vi "SetAttributeViBoolean.vi"(7 "AttributeValue (Off)":bool, 8 "error in (no error)":errorcluster {"code" format="%.0x"}, 9 "AttributeID":u32(ring)=1150001 items=["CHANNEL_AVERAGING"=1150001, "CHANNEL_CORRECTION"=1150003, "CHANNEL_MEASUREMENT_LIMIT_ENABLE"=1150018, "CHANNEL_MEASUREMENT_MARKER_ENABLED"=1150022, "CHANNEL_MEASUREMENT_MARKER_MARKER_TRACK_ENABLED"=1150023, "CHANNEL_MEASUREMENT_SMOOTHING"=1150015, "CHANNEL_MEASUREMENT_TIME_DOMAIN_COUPLING_STATE"=1150136, "CHANNEL_MEASUREMENT_TIME_DOMAIN_GATING_ENABLE"=1150139, "CHANNEL_MEASUREMENT_TIME_DOMAIN_TRANSFORM_ENABLE"=1150146, "CHANNEL_MEASUREMENT_TRACE_ENABLE_TRACE_MAX"=1150182, "CHANNEL_PORT_EXTENSION_STATUS"=1150008, "CHANNEL_SOURCEPOWER_COUPLING"=1150031, "CHANNEL_SWEEP_TIME_AUTO"=1150011, "DISPLAY_ENABLED"=1150036, "GUIDED_CALIBRATION_ADVANCED_E_CAL_AUTO_ORIENTATION"=1150116, "SIMULATE"=1050005, "SYSTEM_POWER_ENABLED"=1150184, "SYSTEM_TRACE_ENABLED"=1150041, "WINDOW_STATE"=1150183, "WINDOW_TITLE_STATE"=1150132], 10 "RepCapIdentifier":string, 11 "instrument handle":refnum<k15>) -> (0 "error out":errorcluster {"code" format="%.0x"}, 3 "instrument handle out":refnum<k15>)   [LabVIEW 2014, in "Agilent NA.lvlib"]
doc: "Sets a Boolean attribute from the instrument driver.\nThe following Attributes are supported:\n\nCHANNEL_AVERAGING\nCHANNEL_CORRECTION\nCHANNEL_MEASUREMENT_LIMIT_ENABLE\nCHANNEL_MEASUREMENT_MARKER_ENABLED\nCHANNEL_MEASUREMENT_MARKER_MARKER_TRACK_ENABLED\nCHANNEL_MEASUREMENT_SMOOTHING\nCHANNEL_MEASUREMENT_TIME_DOMAIN_COUPLING_STATE\nCHANNEL_MEASUREMENT_TIME_DOMAIN_GATING_ENABLE\nCHANNEL_MEASUREMENT_TIME_DOMAIN_TRANSFORM_ENABLE\nCHANNEL_MEASUREMENT_TRACE_ENABLE_TRACE_MAX\nCHANNEL_PORT_EXTENSION_STATUS\nCHANNEL_SOURCEPOWER_COUPLING\nCHANNEL_SWEEP_TIME_AUTO\nDISPLAY_ENABLED\nGUIDED_CALIBRATION_ADVANCED_E_CAL_AUTO_ORIENTATION\nSIMULATE\nSYSTEM_POWER_ENABLED\nSYSTEM_TRACE_ENABLED\nWINDOW_STATE\nWINDOW_TITLE_STATE"
uses:
  Agilent NA.lvlib
  AgNA.dll
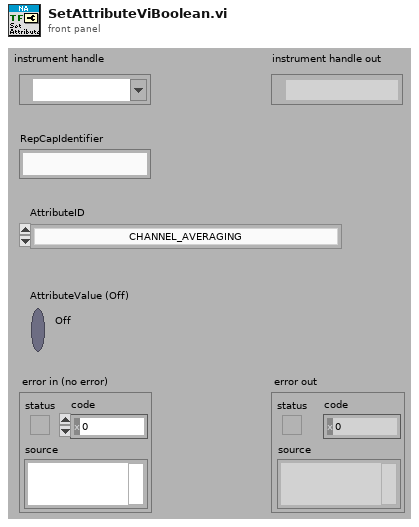
[diagram p1: front panel]
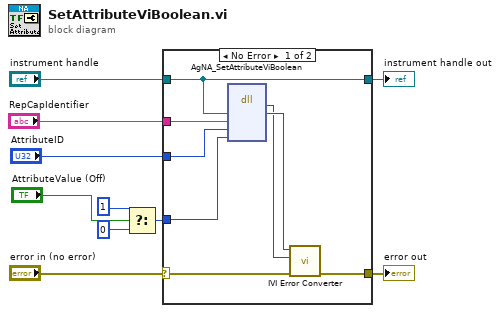
[diagram p0: block diagram]
diagram:
  n1 = Select(t=u16 1, s="AttributeValue (Off)", f=u16 0) -> (s? t:f=w3:u16)
  n2 = case shown="No Error" "error in (no error)" {
    selector: "error in (no error)" -> [w16 w20]
    tunnel: [w15 w20] -> w10
    tunnel: "RepCapIdentifier" -> [w14 _]
    tunnel: "AttributeID" -> [w13 _]
    tunnel: w3 -> [w12 _]
    tunnel: [w11 w19] -> w2
    tunnel: "instrument handle" -> [w11 w19]
    frame No Error {
      n3 = dll-call lib="AgNA**.dll" fn="AgNA_SetAttributeViBoolean"("Vi"=w11, "RepCapIdentifier"=w14, "AttributeID"=w13, "AttributeValue"=w12) -> ("return type"=w17:i32, "Vi"=w18:u32)  [unwired: 6 in, 2 out]
      n4 = call "IVI Error Converter.vi"("error in (no error)"=w16, "IVI error code (0)"=w17, "instrument handle"=w18) -> ("error out"=w15:errorcluster)  [unwired: 7 in, 1 out]
    }
    frame Error {
    }
  }
  "error out" <- w10
  "instrument handle out" <- w2
